vi ".NET Type Builder Marshal String Field.vi"(8 "error in (no error)":errorcluster, 9 ".NET Field Builder":refnum<k24>, 10 "Byte Count":i32) -> (0 "error out":errorcluster, 1 ".NET Field Builder":refnum<k24>)   [LabVIEW 2018, in "TwinCAT ADS.lvclass"]
uses:
  TwinCAT ADS.lvclass
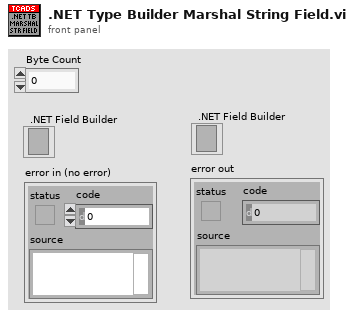
[diagram p1: front panel]
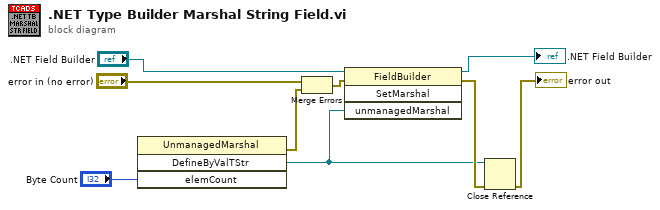
[diagram p0: block diagram]
diagram:
  n1 = invoke class="UnmanagedMarshal" method="DefineByValTStr"("elemCount"="Byte Count") -> (error out=w8:errorcluster, "DefineByValTStr"=w1:refnum<k24>)  [unwired: 3 in, 2 out]
  n2 = Merge Errors("error in (no error)", w8) -> (w9:errorcluster)
  n3 = invoke class="FieldBuilder" method="SetMarshal"(reference=".NET Field Builder", error in=w9, "unmanagedMarshal"=w1) -> (reference out=→".NET Field Builder":refnum<k24>, error out=w7:errorcluster)  [unwired: 1 in, 2 out]
  n4 = Close Reference(reference=w1, error in (no error)=w7) -> (error out=→"error out":errorcluster)
